vi "Read Signed Integer Configuration.vi"(7 "Type":T1, 8 "error in (no error)":errorcluster, 9 "Default If Not Found":i64, 10 "Name":string, 11 "IniFileSection in":refnum<class "IniFileSection.lvclass">) -> (0 "error out":errorcluster, 1 "Not Found?":bool, 2 "Value":i64, 3 "IniFileSection out":refnum<class "IniFileSection.lvclass">)   [LabVIEW 2019, in "IniFileSection.lvclass"]
uses:
  <vilib>/gpm_packages/@cs/Configuration/Source/IniFileSection/IniFileSection.lvclass
  <vilib>/Utility/Data Type/Type Definitions/Data Type.ctl
  <vilib>/gpm_packages/@cs/Configuration/Source/IniFileSection/IniFileSection.lvclass/IniFileSection.ctl
  <vilib>/Utility/config.llb/NI_LVConfig.lvlib
  <vilib>/Utility/Data Type/NI_Data Type.lvlib
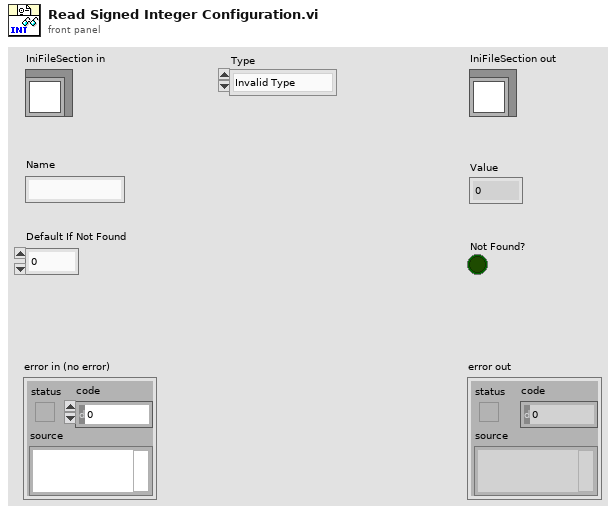
[diagram p1: front panel]
types:
  T1 = typedef "NI_Data Type.lvlib/Data Type.ctl" = enum8{"Invalid Type", "Void", "I8", "I16", "I32", "I64", "U8", "U16", "U32", "U64", "Single Float", "Double Float", "Extended Float", "Single Complex", "Double Complex", "Extended Complex", "Enum U8", "Enum U16", "Enum U32", "Enum U64", "Single Float With Unit", "Double Float With Unit", "Extended Float With Unit", "Single Complex with Unit", "Double Complex with Unit", "Extended Complex with Unit", "Boolean", "String", "Path", "Picture", "Tag", "Array", "Cluster", "Variant", "LV Variant", "Waveform", "Timestamp", "Digital Waveform", "Digital Data", "ExpressData", "Refnum", "External Data", "VI", "Poly VI", "LabVIEW Class Instance", "Fixed Point", "Set Collection", "Map Collection"}
  T2 = typedef "NI_LVConfig.lvlib/Config Data RefNum.ctl" = refnum<k1>
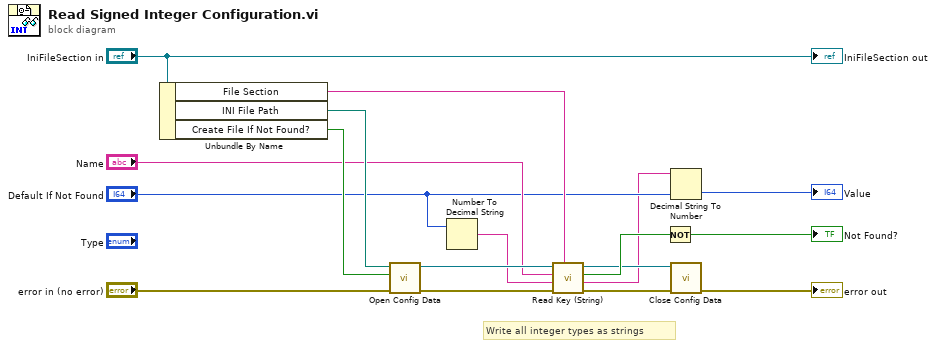
[diagram p0: block diagram]
diagram:
  # "Write all integer types as strings"
  n1 = Unbundle By Name("IniFileSection in") -> ("File Section"=w6:string, "INI File Path"=w14:path, "Create File If Not Found?"=w13:bool)
  n2 = call <vilib>:"Open Config Data.vi"("error in (no error)"="error in (no error)", "create file if necessary (T)"=w13, "configuration file path"=w14) -> ("error out"=w10:errorcluster, "refnum"=w17:T2)  [unwired: 6 in, 1 out]
  n3 = Number To Decimal String(number="Default If Not Found") -> (decimal integer string=w11:string)  [unwired: 1 in]
  n4 = call <vilib>:"Read Key (String).vi"("section"=w6, "error in (no error)"=w10, "default value"=w11, "key"="Name", "refnum"=w17) -> ("error out"=w9:errorcluster, "value"=w2:string, "found?"=w12:bool, "refnum out"=w8:T2)  [unwired: 3 in]
  n5 = Not(x=w12) -> (.not. x?=→"Not Found?":bool)
  n6 = Decimal String To Number(string=w2, default (0L)="Default If Not Found") -> (number=→"Value":i64)  [unwired: 1 in, 1 out]
  n7 = call <vilib>:"Close Config Data.vi"("error in (no error)"=w9, "refnum"=w8) -> ("error out"=→"error out":errorcluster)  [unwired: 8 in, 1 out]
  "IniFileSection out" <- "IniFileSection in"
